vi "Handle Menu Activation.vi"(8 "error in":errorcluster, 10 "Menu in":refnum<k9>, 11 "Configuration In":T1) -> (0 "error out":errorcluster)   [LabVIEW 2013, in "LVTM.lvlib"]
uses:
  LVTM.lvlib
  Controls_LVTM/LVTM_Config_Info.ctl
  Controls_LVTM/View.ctl
  Controls_LVTM/SharedDataDVR.ctl
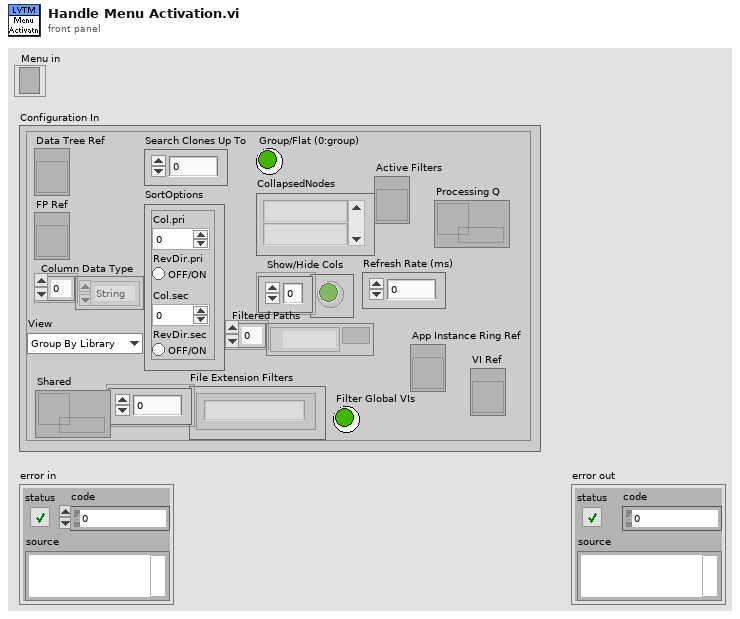
[diagram p1: front panel]
types:
  T1 = typedef "LVTM.lvlib/LVTM_Config_Info.ctl" = cluster{"Data Tree Ref":refnum<vi>, "FP Ref":refnum<vi>, "Column Data Type":enum16{"String", "Numeric"}[], "Search Clones Up To":i32, "SortOptions":cluster{"Col.pri":i32, "RevDir.pri":bool, "Col.sec":i32, "RevDir.sec":bool}, "Group/Flat (0:group)":bool, "CollapsedNodes":string[], "Show/Hide Cols":bool[], "Filtered Paths":path[], "View":T2, "File Extension Filters":string[], "Filter Global VIs":bool, "Shared":refnum<data-value>, "Active Filters":refnum<vi>, "Refresh Rate (ms)":i32, "App Instance Ring Ref":refnum<vi>, "Processing Q":refnum<queue>, "VI Ref":refnum<vi>}
  T2 = typedef "LVTM.lvlib/View.ctl" = enum16{"Group By Library", "Group By Folder", "Flat List"}
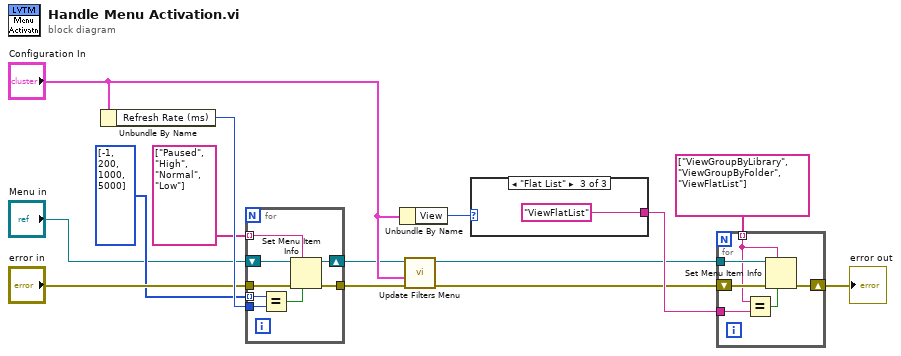
[diagram p0: block diagram]
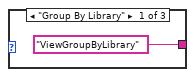
[diagram p2: hidden frame]
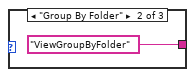
[diagram p3: hidden frame]
diagram:
  n1 = Unbundle By Name("Configuration In") -> ("Refresh Rate (ms)"=w14:i32)
  n2 = for {
    tunnel: string[] ["Paused", "High", "Normal", "Low"] -> [w21] mode=indexing
    tunnel: w14 -> [w20]
    tunnel: i32[] [-1, 200, 1000, 5000] -> [w18] mode=indexing
    tunnel: "error in" -> [w17]
    tunnel: [w16] -> w5
    shift-right: [w15] -> w6
    shift-left: "Menu in" -> [w22]
    n3 = Equal?(x=w18, y=w20) -> (x = y?=w19:bool)
    n4 = Set Menu Item Info(6:w19, 7:w21, 8:w17, 11:w22) -> (0:w16:errorcluster, 3:w15:refnum<k9>)  [unwired: 3 in]
  }
  n5 = Unbundle By Name("Configuration In") -> ("View"=w7:T2)
  n6 = call "Update Filters Menu.vi"("error in"=w5, "ConfigInfo in"="Configuration In", "Menu in"=w6) -> ("error out"=w10:errorcluster, "Menu out"=w8:refnum<k9>)  [unwired: 7 in]
  n7 = case shown="\"Flat List\"" w7 {
    tunnel: ["ViewGroupByLibrary" ("item tag") "ViewGroupByFolder" ("item tag") "ViewFlatList" ("item tag")] -> w12
    frame "Group By Library" {
    }
    frame "Group By Folder" {
    }
    frame "Flat List" {
    }
  }
  n8 = for {
    tunnel: w8 -> [w31]
    tunnel: string[] ["ViewGroupByLibrary", "ViewGroupByFolder", "ViewFlatList"] -> [w28] mode=indexing
    shift-right: [w30] -> w9
    shift-left: w10 -> [w29]
    tunnel: w12 -> [w27]
    n9 = Equal?(x=w28, y=w27) -> (x = y?=w26:bool)
    n10 = Set Menu Item Info(6:w26, 7:w28, 8:w29, 11:w31) -> (0:w30:errorcluster)  [unwired: 3 in, 1 out]
  }
  "error out" <- w9
